vi "PluginExample.vi"   [LabVIEW 2016]
doc: "This Example shows the add functionality of the menu builder. Each plugin class define's what it's menu should look like. When the plugin is loaded into memory at runtime, it's menu item is added to the menu."
uses:
  <userlib>/_MGI/Menu Building/Example/Plugin/MGI_Plugin.lvclass
  <userlib>/_MGI/Menu Building/MenuItem/MenuSeparatorItem/MGI_MenuSeparatorItem.lvclass
  C:/Program Files (x86)/National Instruments/LabVIEW 2016/user.lib/_MGI/Menu Building/MenuItem/MGI_MenuItem.lvclass
  <userlib>/_MGI/Menu Building/MenuItem/VIItem/MGI_VIItem.lvclass
  <userlib>/_MGI/Menu Building/MenuTypes/Vi/MGI_VI.lvclass
  C:/Program Files (x86)/National Instruments/LabVIEW 2016/user.lib/_MGI/Menu Building/MenuTypes/MGI_Menu.lvclass
  <userlib>/_MGI/Menu Building/MenuItem/VIItem/VIItem.vi
  <userlib>/_MGI/Menu Building/MenuItem/MenuItem.vi
  <userlib>/_MGI/Menu Building/MenuItem/MenuSeparatorItem/MenuSeparatorItem.vi
  <userlib>/_MGI/Menu Building/MenuItem/Write Sub-Menus.vi
  <userlib>/_MGI/Menu Building/MenuTypes/Vi/VI.vi
  <userlib>/_MGI/Menu Building/MenuItemStatusChange/Read MenuItem.vi
  <userlib>/_MGI/Menu Building/MenuItem/Read Full Tag.vi
  <userlib>/_MGI/Menu Building/MenuItem/MGI_MenuItem.lvclass
  <userlib>/_MGI/Menu Building/MenuTypes/MGI_Menu.lvclass
  <userlib>/_MGI/Menu Building/MenuItemStatusChange/MGI_MenuItemStatusChange.lvclass
panel:
  # "Use the Runtime Menu to add, configure, and run plugins."
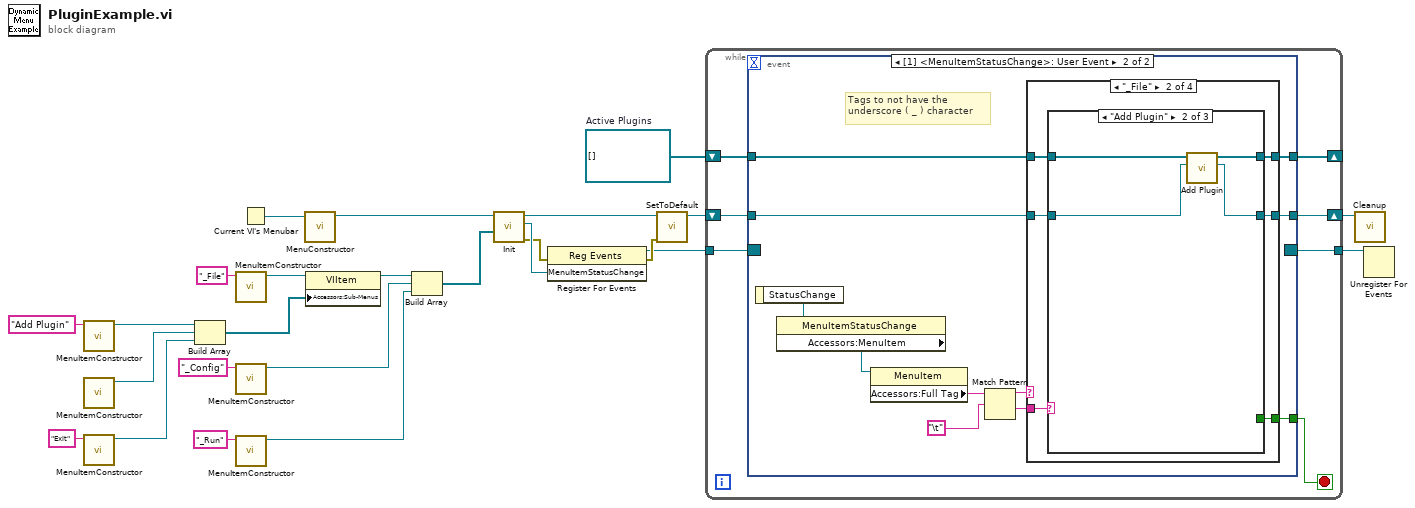
[diagram p0: block diagram]
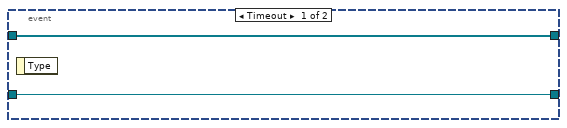
[diagram p2: hidden frame]
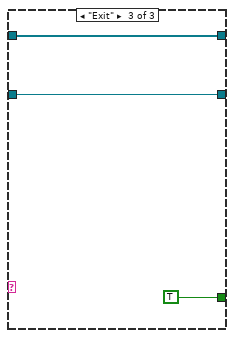
[diagram p5: hidden frame]
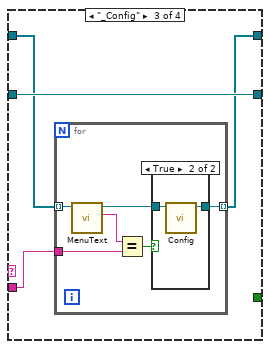
[diagram p6: hidden frame]
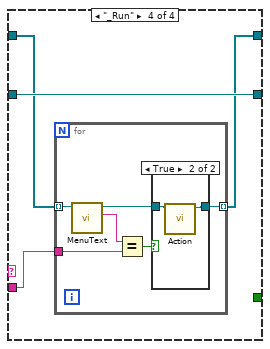
[diagram p8: hidden frame]
diagram:
  w4 = refnum<class "MGI_Plugin.lvclass">[] []  # Active Plugins
  n1 = call-poly <userlib>:"MenuItemConstructor.vi"("Text"="Add Plugin") -> ("MenuItem"=w21:refnum<data-value>)  [unwired: 9 in, 1 out]
  n2 = call-poly <userlib>:"MenuItemConstructor.vi"() -> ("MenuSeparatorItem"=w19:refnum<data-value>)  [unwired: 10 in, 1 out]
  n3 = call-poly <userlib>:"MenuItemConstructor.vi"("Text"="Exit") -> ("MenuItem"=w18:refnum<data-value>)  [unwired: 9 in, 1 out]
  n4 = Build Array(w21, w19, w18) -> (w20:refnum<data-value>[])
  n5 = call-poly <userlib>:"MenuItemConstructor.vi"("Text"="_File") -> ("VIItem Item"=w1:refnum<data-value>)  [unwired: 9 in, 1 out]
  n6 = call-poly <userlib>:"MenuItemConstructor.vi"("Text"="_Config") -> ("MenuItem"=w6:refnum<data-value>)  [unwired: 9 in, 1 out]
  n7 = call-poly <userlib>:"MenuItemConstructor.vi"("Text"="_Run") -> ("MenuItem"=w5:refnum<data-value>)  [unwired: 9 in, 1 out]
  n8 = Current VI's Menubar() -> (w9:refnum<k9>)
  n9 = call-poly <userlib>:"MenuConstructor.vi"("menu reference"=w9) -> ("VI"=w15:refnum<class "MGI_VI.lvclass">)  [unwired: 9 in, 1 out]
  n10 = property class="VIItem"(reference=w1, "Accessors:Sub-Menus"=w20) -> (reference out=w17:refnum<data-value>)  [unwired: 1 in, 1 out]
  n11 = Build Array(w17, w6, w5) -> (w7:refnum<data-value>[])
  n12 = call-dynamic "Init.vi"("Menu Items"=w7, "Menu in"=w15) -> ("error out"=w12:errorcluster, "MenuItemStatusChange"=w14:refnum<user-event>, "Menu out"=w16:refnum<class "MGI_VI.lvclass">)  [unwired: 7 in]
  n13 = register-events(error in=w12, w14) -> (reference out=w10:refnum<event-registration>, error out=w13:errorcluster)  [unwired: 1 in]
  n14 = call-dynamic "SetToDefault.vi"("error in (no error)"=w13, "Menu in"=w16) -> ("Menu out"=w11:refnum<class "MGI_VI.lvclass">)  [unwired: 8 in, 1 out]
  n15 = while {
    shift-right: [w31] -> w8
    shift-left: w11 -> [w32]
    tunnel: w10 -> [w30]
    shift-right: [w28] -> _
    shift-left: w4 -> [w29]
    tunnel: [w26] -> w3
    stop <- w27 stop-if-true
    n16 = event shown="[1] <MenuItemStatusChange>: User Event" {
      selector: w30 -> [_ _]
      dyn-events: [_ _] -> w26
      timeout: _ -> [_ _]
      tunnel: w32 -> [w34 w42]
      tunnel: [w34 w41] -> w31
      tunnel: w29 -> [w33 w43]
      tunnel: [w33 w40] -> w28
      tunnel: [_ w39] -> w27
      event Timeout {
        n17 = event-data() -> ()  [unwired: 1 in, 1 out]
      }
      event User Event {
        # "Tags to not have the underscore ( _ ) character"
        n18 = event-data() -> ("StatusChange"=w45:refnum<class "MGI_MenuItemStatusChange.lvclass">)  [unwired: 1 in]
        n19 = property class="MenuItemStatusChange"(reference=w45) -> ("Accessors:MenuItem"=w44:refnum<data-value>)  [unwired: 1 in, 2 out]
        n20 = property class="MenuItem"(reference=w44) -> ("Accessors:Full Tag"=w38:string)  [unwired: 1 in, 2 out]
        n21 = Match Pattern(string=w38, regular expression="\t") -> (before substring=w37:string, after substring=w36:string)  [unwired: 1 in, 2 out]
        n22 = case shown="\"_File\"" w37 {
          tunnel: w43 -> [w47 w53 w65 w78]
          tunnel: w42 -> [w46 w52 w66 w79]
          tunnel: [w46 w51 w66 w79] -> w41
          tunnel: [w47 w50 w63 w76] -> w40
          tunnel: [_ w49 _ _] -> w39
          tunnel: w36 -> [_ w48 w64 w77]
          frame Default {
          }
          frame "_File" {
            n23 = case shown="\"Add Plugin\"" w48 {
              tunnel: w53 -> [w55 w59 w61]
              tunnel: w52 -> [w54 w57 w62]
              tunnel: [w54 w56 w62] -> w51
              tunnel: [w55 w58 w61] -> w50
              tunnel: [_ _ TRUE] -> w49
              frame Default {
              }
              frame "Add Plugin" {
                n24 = call <userlib>:"Add Plugin.vi"("Menu in"=w57, "Active Plugins in"=w59) -> ("Menu out"=w56:refnum<class "MGI_VI.lvclass">, "Active Plugins out"=w58:refnum<class "MGI_Plugin.lvclass">[])  [unwired: 8 in]
              }
              frame "Exit" {
              }
            }
          }
          frame "_Config" {
            n25 = for {
              tunnel: w65 -> [w72] mode=indexing
              tunnel: w64 -> [w70]
              tunnel: [w67] -> w63 mode=indexing
              n26 = call-dynamic "MenuText.vi"("MGI_Plugin.lvclass"=w72) -> ("Menu Text"=w71:string, "MGI_Plugin.lvclass"=w68:refnum<class "MGI_Plugin.lvclass">)  [unwired: 8 in, 1 out]
              n27 = Equal?(x=w71, y=w70) -> (x = y?=w69:bool)
              n28 = case shown="True" w69 {
                tunnel: w68 -> [w73 w75]
                tunnel: [w73 w74] -> w67
                frame False {
                }
                frame True {
                  n29 = call-dynamic "Config.vi"("MGI_Plugin.lvclass"=w75) -> ("MGI_Plugin.lvclass"=w74:refnum<class "MGI_Plugin.lvclass">)  [unwired: 9 in, 1 out]
                }
              }
            }
          }
          frame "_Run" {
            n30 = for {
              tunnel: w78 -> [w85] mode=indexing
              tunnel: w77 -> [w83]
              tunnel: [w80] -> w76 mode=indexing
              n31 = call-dynamic "MenuText.vi"("MGI_Plugin.lvclass"=w85) -> ("Menu Text"=w84:string, "MGI_Plugin.lvclass"=w81:refnum<class "MGI_Plugin.lvclass">)  [unwired: 8 in, 1 out]
              n32 = Equal?(x=w84, y=w83) -> (x = y?=w82:bool)
              n33 = case shown="True" w82 {
                tunnel: w81 -> [w86 w88]
                tunnel: [w86 w87] -> w80
                frame False {
                }
                frame True {
                  n34 = call-dynamic "Action.vi"("MGI_Plugin.lvclass"=w88) -> ("MGI_Plugin.lvclass"=w87:refnum<class "MGI_Plugin.lvclass">)  [unwired: 9 in, 1 out]
                }
              }
            }
          }
        }
      }
    }
  }
  n35 = call-dynamic "Cleanup.vi"("VI"=w8) -> ()  [unwired: 10 in, 1 out]
  n36 = Unregister For Events(event registration refnum=w3) -> ()  [unwired: 1 in, 1 out]
